vi "from string.vi"(8 "error in":errorcluster, 9 "data":string, 10 "version":string, 11 "TEC configuration in":refnum<class "TEC configuration.lvclass">) -> (0 "error out":errorcluster, 3 "TEC configuration out":refnum<class "TEC configuration.lvclass">)   [LabVIEW 2013, in "TEC configuration.lvclass"]
doc: "Provides an interface for loading a module configuration from a file or other serialized data source. It is recommended that all children of this class store data in two sets--data required for its own initialization, and any data required for parent initialization--and that each implementation uses the <b>Call Parent Method</b> primitive to de-serialize parent information. As a result, it is expected that every module configuration class calls <b>component configuration.lvclass:From String.vi</b>."
uses:
  TEC configuration.lvclass
  <vilib>/NI/Tag Bus Module Framework/channel/TBM channel.lvclass
  <vilib>/NI/Tag Bus Module Framework/module configuration/TBM module configuration.lvclass
  TEC configuration.lvclass/TEC configuration.ctl
  <vilib>/NI/Configuration Framework/serializable configuration/NISE_CEF_serializable configuration.lvclass
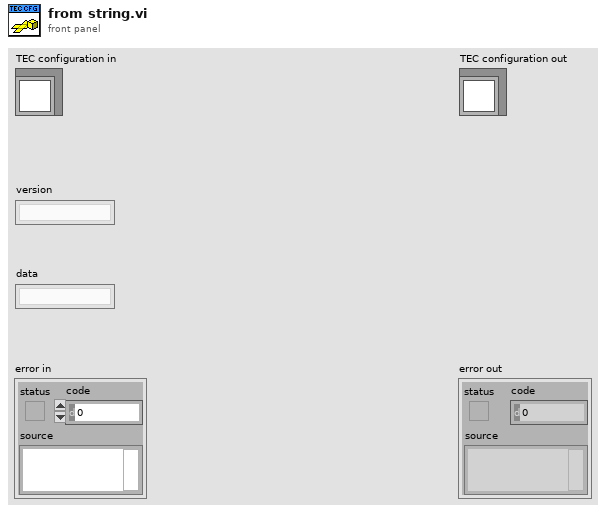
[diagram p1: front panel]
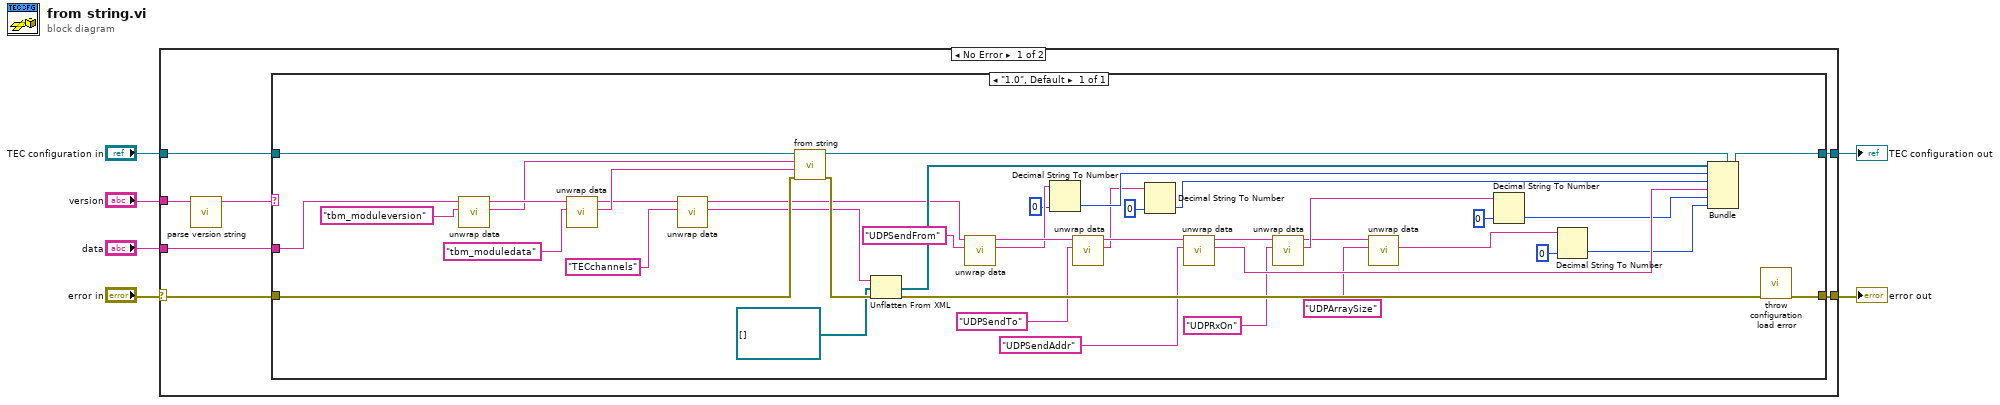
[diagram p0: block diagram]
diagram:
  n1 = case shown="No Error" "error in" {
    selector: "error in" -> [w7 w56]
    tunnel: "data" -> [w13 _]
    tunnel: "TEC configuration in" -> [w12 w55]
    tunnel: [w11 w55] -> w5
    tunnel: [w10 w56] -> w4
    tunnel: "version" -> [w9 _]
    frame No Error {
      n2 = call <vilib>:"parse version string.vi"("full version"=w9) -> ("major.minor version"=w8:string)  [unwired: 7 in, 3 out]
      n3 = case shown="\"1.0\", Default" w8 {
        tunnel: w13 -> [w49]
        tunnel: w7 -> [w48]
        tunnel: w12 -> [w54]
        tunnel: [w43] -> w11
        tunnel: [w51] -> w10
        frame "1.0", Default {
          n4 = call <vilib>:"unwrap data.vi"("identifier"="tbm_moduleversion" ("additional identifier"), "data to unwrap"=w49) -> ("unwrapped data"=w44:string, "remaining string"=w50:string)  [unwired: 8 in]
          n5 = call <vilib>:"unwrap data.vi"("identifier"="tbm_moduledata" ("additional identifier"), "data to unwrap"=w50) -> ("unwrapped data"=w46:string, "remaining string"=w39:string)  [unwired: 8 in]
          n6 = call <vilib>:"unwrap data.vi"("identifier"="TECchannels" ("additional identifier"), "data to unwrap"=w39) -> ("unwrapped data"=w37:string, "remaining string"=w33:string)  [unwired: 8 in]
          n7 = call-parent "from string.vi"("error in"=w48, "data"=w46, "version"=w44, "module configuration in"=w54) -> ("error out"=w52:errorcluster, "module configuration out"=w53:refnum<class "TEC configuration.lvclass">)  [unwired: 6 in]
          n8 = Unflatten From XML(xml string=w37, type=refnum<class "TBM channel.lvclass">[] [] ("channels"), error in (no error)=w52) -> (value=w40:refnum<class "TBM channel.lvclass">[], error out=w42:errorcluster)
          n9 = call <vilib>:"unwrap data.vi"("identifier"="UDPSendFrom" ("additional identifier"), "data to unwrap"=w33) -> ("unwrapped data"=w31:string, "remaining string"=w35:string)  [unwired: 8 in]
          n10 = Decimal String To Number(string=w31, default (0L)=u16 0 ("default (0 I32)")) -> (number=w24:u16)  [unwired: 1 in, 1 out]
          n11 = call <vilib>:"unwrap data.vi"("identifier"="UDPSendTo" ("additional identifier"), "data to unwrap"=w35) -> ("unwrapped data"=w23:string, "remaining string"=w36:string)  [unwired: 8 in]
          n12 = Decimal String To Number(string=w23, default (0L)=u16 0 ("default (0 I32)")) -> (number=w25:u16)  [unwired: 1 in, 1 out]
          n13 = call <vilib>:"unwrap data.vi"("identifier"="UDPSendAddr" ("additional identifier"), "data to unwrap"=w36) -> ("unwrapped data"=w27:string, "remaining string"=w34:string)  [unwired: 8 in]
          n14 = call <vilib>:"unwrap data.vi"("identifier"="UDPRxOn" ("additional identifier"), "data to unwrap"=w34) -> ("unwrapped data"=w22:string, "remaining string"=w17:string)  [unwired: 8 in]
          n15 = call <vilib>:"unwrap data.vi"("identifier"="UDPArraySize" ("additional identifier"), "data to unwrap"=w17) -> ("unwrapped data"=w16:string)  [unwired: 8 in, 1 out]
          n16 = Decimal String To Number(string=w22, default (0L)=u16 0 ("default (0 I32)")) -> (number=w26:u16)  [unwired: 1 in, 1 out]
          n17 = Decimal String To Number(string=w16, default (0L)=u16 0 ("default (0 I32)")) -> (number=w15:u16)  [unwired: 1 in, 1 out]
          n18 = Bundle(cluster=w53, w40, w24, w25, w27, w26, w15) -> (w43:refnum<class "TEC configuration.lvclass">)
          n19 = call <vilib>:"throw configuration load error.vi"("error in"=w42) -> ("error out"=w51:errorcluster)  [unwired: 10 in]
        }
      }
    }
    frame Error {
    }
  }
  "error out" <- w4
  "TEC configuration out" <- w5
